vi "Class Not Found.vi"(7 "error source vi name":string, 8 "error in (no error)":errorcluster, 10 "class path":path, 11 "Component Loader in":refnum<class "Component Loader.lvclass">) -> (0 "error out":errorcluster, 3 "Component Loader out":refnum<class "Component Loader.lvclass">)   [LabVIEW 2017, in "DSF Core.lvlib" / "Component Loader.lvclass"]
uses:
  Component Loader.lvclass
  Errors.ctl
  <vilib>/NI/Memory Manager/Static Error Handling.lvlib
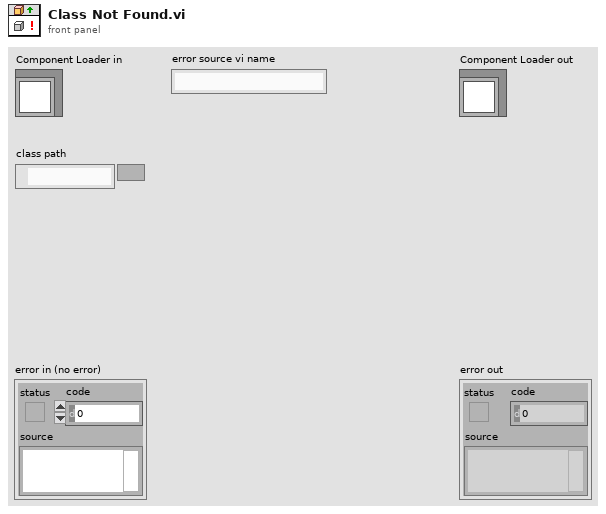
[diagram p1: front panel]
types:
  T1 = typedef "DSF Core.lvlib/Component Loader.lvclass/Errors.ctl" = enum16{"Component Directory Not Found", "Component Not Found", "Class Not Found"}
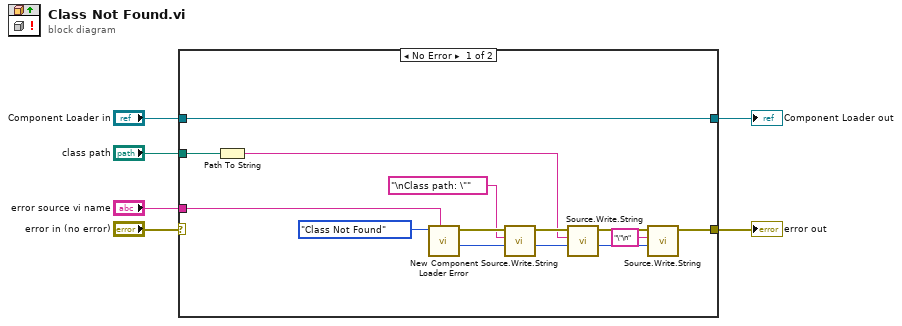
[diagram p0: block diagram]
diagram:
  n1 = case shown="No Error" "error in (no error)" {
    selector: "error in (no error)" -> [_ w22]
    tunnel: [w9 w22] -> w5
    tunnel: "error source vi name" -> [w19 _]
    tunnel: "Component Loader in" -> [w18 w21]
    tunnel: [w18 w21] -> w2
    tunnel: "class path" -> [w8 _]
    frame No Error {
      n2 = Path To String(path=w8) -> (string=w7:string)
      n3 = call "New Component Loader Error.vi"("error source vi name"=w19, "error"=Errors."Class Not Found") -> ("new offset"=w16:i32, "error out"=w17:errorcluster)  [unwired: 8 in]
      n4 = call <vilib>:"Source.Write.String.vi"("offset"=w16, "string"="\nClass path: \"", "error in"=w17) -> ("new offset"=w15:i32, "error out"=w14:errorcluster)  [unwired: 7 in]
      n5 = call <vilib>:"Source.Write.String.vi"("offset"=w15, "string"=w7, "error in"=w14) -> ("new offset"=w11:i32, "error out"=w12:errorcluster)  [unwired: 7 in]
      n6 = call <vilib>:"Source.Write.String.vi"("offset"=w11, "string"="\"\n", "error in"=w12) -> ("error out"=w9:errorcluster)  [unwired: 7 in, 1 out]
    }
    frame Error {
    }
  }
  "error out" <- w5
  "Component Loader out" <- w2
